vi "CHOPout.vi"(1 "Async ?":bool, 5 "IN VARIANT":variant, 7 "Ip":string, 9 "Name in":string, 11 "error in (no error)":errorcluster) -> (10 "Operation Ok":bool, 15 "error out":errorcluster)   [LabVIEW 2015]
uses:
  CHOPS_COUPLE_separator_string.ctl
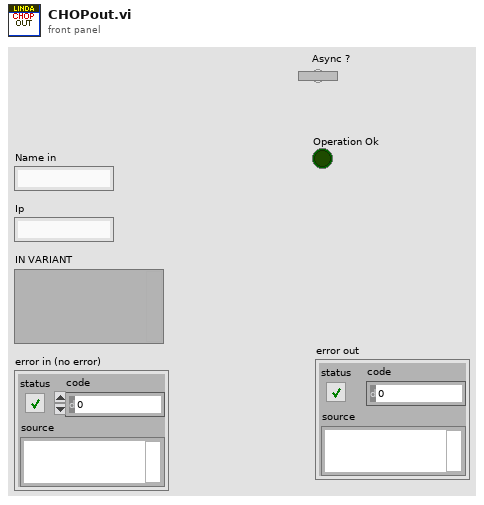
[diagram p1: front panel]
types:
  T1 = typedef "CHOPS_COUPLE_separator_string.ctl" = string
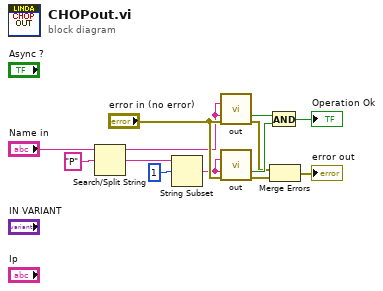
[diagram p0: block diagram]
diagram:
  n1 = Search/Split String(string="Name in", search string/char (-)=T1 "P") -> (substring before match=w1:string, match + rest of string=w12:string)  [unwired: 1 in, 1 out]
  n2 = String Subset(string=w12, offset (0)=1) -> (substring=w2:string)  [unwired: 1 in]
  n3 = call "out.vi"("IN VARIANT"=w1, "Name in"=w1, "error in (no error)"="error in (no error)") -> ("Operation Ok"=w9:bool, "error out"=w5:errorcluster)  [unwired: 11 in]
  n4 = call "out.vi"("IN VARIANT"=w2, "Name in"=w2, "error in (no error)"="error in (no error)") -> ("Operation Ok"=w8:bool, "error out"=w4:errorcluster)  [unwired: 11 in]
  n5 = And(x=w9, y=w8) -> (x .and. y?=→"Operation Ok":bool)
  n6 = Merge Errors(w5, w4) -> (→"error out":errorcluster)
